vi "PH_gentec_P-Link.panel.vi"(0 "object ref":refnum<vi>, 5 "error in (no error)":errorcluster) -> (19 "error out":errorcluster)   [LabVIEW 2014, in "PH_gentec_P-Link.lvlib"]
doc: "By this VI apowermeter can be operated. \n\nThe panel is divided into the Tab Control which contains three pages and the most important elements.\nThe 1st page of the Tab Control contains the general information Range, Trigger Level, Scaling Factor (the user can set these values), Uncorrected Value and Serial Number (these are indicators). \nThe 2nd page contains everything relevant for the Statistics Mode of the powermeter. Here you can Start/Stop the statistic data collection, set the Number of Pulses, Percentage of Pulses and the Number of Samples. The Cluster 'Statistic Data' views the evaluated statistic data.\nThe 3rd page contains the rarely needed status-information of the powermeter. The string views data like Active Sensitivity, Offset, Resolution and so on.\n\nBelow the Tab Control you can see: \n - Current Value views the value that is currently being displayed on the device's screen. The correct unit is appended.\n - Powermeter views the Device State: blue means no info\n darkgreen means off\n lightgreen means operating\n yellow means error detected\n - EXIT closes the front panel (GUI), while\n - Delete Instance disconnects and removes the instance from the PCS.\n\n\nLicense Agreement for this software:\n\nCopyright (C)\nGesellschaft für Schwerionenforschung, GSI\nPlanckstr. 1\n64291 Darmstadt\nGermany\n\nContact: D.Beck@gsi.de \n\nThis program is free software; you can redistribute it and/or modify it under the terms of the GNU General Public License as published by the Free Software Foundation; either version 2 of the license, or (at your option) any later version.\n\nThis program is distributed in the hope that it will be useful, but WITHOUT ANYW ARRANTY; without even the implied warranty of MERCHANTABILITY or FITNESS FOR A PARTICULAR PURPOSE. See the GNU General License for more details (http://www.gnu.org).\n\nGesellschaft für Schwerionenforschung, GSI\nPlanckstr. 1, 64291 Darmstadt, Germany\nFor all questions and ideas contact: M.Richter@gsi.de, H.Brand@gsi.de or D.Beck@gsi.de.\nLast update: 18-DEC-2002"
uses:
  PH_gentec_P-Link.lvlib
  PH_Basics/PH_StatusHandler/PH_StatusHandler.GUI element.ctl
  PH_Basics/PH_Powermeter_BaseClass/PH_Powermeter_BaseClass.Connection.ctl
  PH_Basics/PH_Powermeter_BaseClass/PH_Powermeter_BaseClass.State.ctl
  PH_Basics/PH_Powermeter_BaseClass/PH_Powermeter_BaseClass.Head Attributes.ctl
  PH_gentec_P-Link.Head Settings.ctl
  instr.lib/Gentec-M-Link/Driver/Type Defs/gentec-M-Link.Measurement Mode.ctl
  instr.lib/Gentec-M-Link/Driver/Type Defs/gentec-M-Link.Trigger Polarity.ctl
  instr.lib/Gentec-M-Link/Driver/Type Defs/gentec-M-Link.Trigger Source.ctl
  instr.lib/Gentec-M-Link/Driver/Type Defs/gentec-M-Link.Waveform Averages.ctl
  PH_Basics/PH_Powermeter_BaseClass/PH_Powermeter_BaseClass.Energy.ctl
  PH_Basics/PH_Powermeter_BaseClass/PH_gentec_BaseClass.Head Settings.ctl
  PH_Basics/PH_Powermeter_BaseClass/PH_Powermeter_BaseClass.GUI Refs.ctl
  CS_Core/CSObj/CSObj.lvlib
  PH_Basics/PH_Common/PH_Common.lvlib
  CS_Core/CSSystem/CSSystemLib/CSSystemLib.lvlib
  PH_Basics/PH_Class/PH_Class.lvlib
  PH_Basics/PH_Powermeter_BaseClass/PH_Powermeter_BaseClass.lvlib
  instr.lib/Gentec-M-Link/gentec-M-Link - Driver.lvlib
  PH_Basics/PH_StatusHandler/PH_StatusHandler.lvlib
panel:
  in  "Tab Control":enum32{"Main", "Sets", "Information"}(tab)
  out "Power":T1={"current Value"=0.0, "unscaled"=0.0, "Scaling Factor"=1.0} {"unscaled" format="%#_6p"; "current Value" format="%#.1p"}
  out "Power evolution":dbl(graph)
  in  "Scaling Factor":dbl=1.0
  in  "Continuous":bool
  in  "get one Value":bool
  in  "Averages":T2 items=["None", "2", "4", "8", "16", "32", "64", "128"]
  in  "Range":u32(ring) items=["Scale 1", "Scale 2", "Scale 3"]
  in  "Set Auto Range":bool
  in  "Wavelength":u32 caption="nm"
  in  "Trigger Source":T3 items=["Internal", "External"]
  in  "Trigger Polarity":T4 items=["Falling Edge", "Rising Edge"]
  in  "Trigger Level":dbl caption="%"
  out "Current Settings":T5={"Trigger Level"=0.0, "Wavelength"=1, "Range"=0}
  out "Wanted Settings":T5={"Trigger Level"=0.0, "Wavelength"=1, "Range"=0}
  out "Wanted Head Settings":T6 {"Waveform Averages" items=["None", "2", "4", "8", "16", "32", "64", "128"]; "Trigger Source" items=["Internal", "External"]; "Trigger Polarity" items=["Falling Edge", "Rising Edge"]; "Measurement Mode" items=["other Mode", "Energymode"]}
  out "Current Head Settings":T6 {"Waveform Averages" items=["None", "2", "4", "8", "16", "32", "64", "128"]; "Trigger Source" items=["Internal", "External"]; "Trigger Polarity" items=["Falling Edge", "Rising Edge"]; "Measurement Mode" items=["other Mode", "Energymode"]}
  out "Connection":T8
  out "VISA resource":refnum<visa-resource-name>
  out "Head Attributes":T10={"Instrument Type"="---", "Head Version"="---", "Head Name"="---", "Serial Number"="---", "Firmware"="---", "Sensor Type"="---", "MinimumRange"=0, "Maximum Range"=0, "Min Wavelength"=-1, "Max Wavelength"=-1}
  out "PSDB Status":u32(colorbox)=6618880 caption="PSDB"
  out "Status":T11 caption="Powermeter"
  in  "Delete":bool
  in  "Exit":bool
  # "PCS"
  # "3.40"
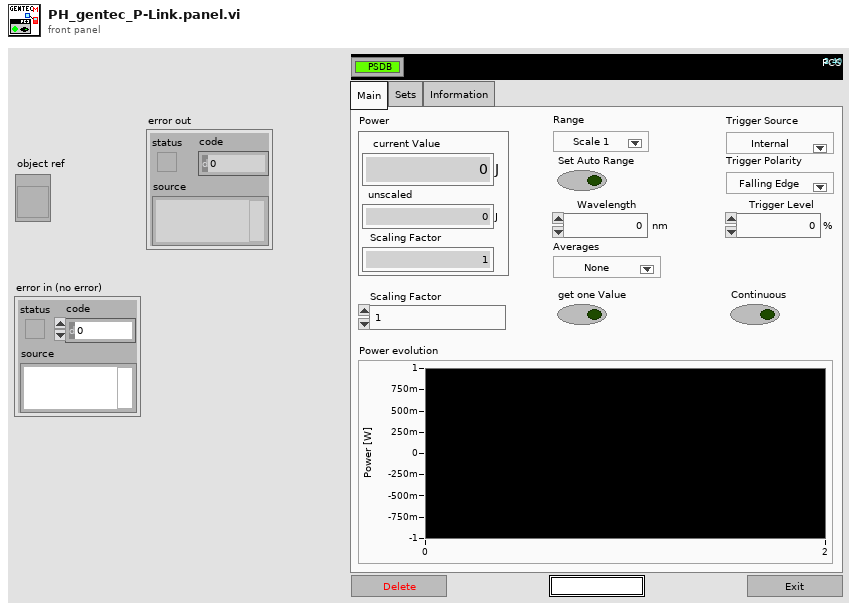
[diagram p1: front panel]
types:
  T1 = typedef "PH_Powermeter_BaseClass.lvlib/PH_Powermeter_BaseClass.Energy.ctl" = cluster{"current Value":dbl, "unscaled":dbl, "Scaling Factor":dbl}
  T2 = typedef "gentec-M-Link - Driver.lvlib/gentec-M-Link.Waveform Averages.ctl" = u16
  T3 = typedef "gentec-M-Link - Driver.lvlib/gentec-M-Link.Trigger Source.ctl" = u16
  T4 = typedef "gentec-M-Link - Driver.lvlib/gentec-M-Link.Trigger Polarity.ctl" = u16
  T5 = typedef "PH_Powermeter_BaseClass.lvlib/PH_gentec_BaseClass.Head Settings.ctl" = cluster{"Trigger Level":dbl, "Wavelength":u32, "Range":u32}
  T6 = typedef "PH_gentec_P-Link.lvlib/PH_gentec_P-Link.Head Settings.ctl" = cluster{"Measurement Mode":T7, "Enable Anticipation":bool, "Set Auto Range":bool, "Block Signal":bool, "Set Head Attenuator":bool, "Enable SSE":bool, "Trigger Polarity":T4, "Trigger Source":T3, "Waveform Averages":T2, "Set Zero":i32, "Current Measurement":i32, "Start Data Flow":bool}
  T7 = typedef "gentec-M-Link - Driver.lvlib/gentec-M-Link.Measurement Mode.ctl" = u16
  T8 = typedef "PH_Powermeter_BaseClass.lvlib/PH_Powermeter_BaseClass.Connection.ctl" = cluster{"failed checks":i8, "Timeout":bool, "Data read":string, "Failure":bool, "Error":bool, "State":T9}
  T9 = typedef "PH_Powermeter_BaseClass.lvlib/PH_Powermeter_BaseClass.State.ctl" = enum32{"off", "operating", "opened", "checked", "connected", "Sets to change", "running"}
  T10 = typedef "PH_Powermeter_BaseClass.lvlib/PH_Powermeter_BaseClass.Head Attributes.ctl" = cluster{"Instrument Type":string, "Head Version":string, "Head Name":string, "Serial Number":string, "Firmware":string, "Sensor Type":string, "MinimumRange":u32, "Maximum Range":u32, "Min Wavelength":i32, "Max Wavelength":i32}
  T11 = typedef "PH_StatusHandler.lvlib/PH_StatusHandler.GUI element.ctl" = u16
  T12 = typedef "PH_Powermeter_BaseClass.lvlib/PH_Powermeter_BaseClass.GUI Refs.ctl" = cluster{"Head Attributes":refnum<vi>, "Energy":refnum<vi>, "Connection":refnum<vi>, "VISA Resource":refnum<vi>, "Energy evolution":refnum<vi>, "Scaling Factor":refnum<vi>, "Range":refnum<vi>, "Wavelength":refnum<vi>, "Trigger Level":refnum<vi>, "Wanted Settings":refnum<vi>, "Current Settings":refnum<vi>}
  T13 = typedef "PH_gentec_P-Link.lvlib/PH_gentec_P-Link.i attribute.ctl" = cluster{"GUI References":cluster{"Wanted Head Settings":refnum<vi>, "Current Head Settings":refnum<vi>, "Set Auto Range":refnum<vi>, "Trigger Polarity":refnum<vi>, "Trigger Source":refnum<vi>, "Waveform Averages":refnum<vi>, "Continuous":refnum<vi>, "get one Value":refnum<vi>}, "Wanted Head Settings":T6, "Current Head Settings":T6}
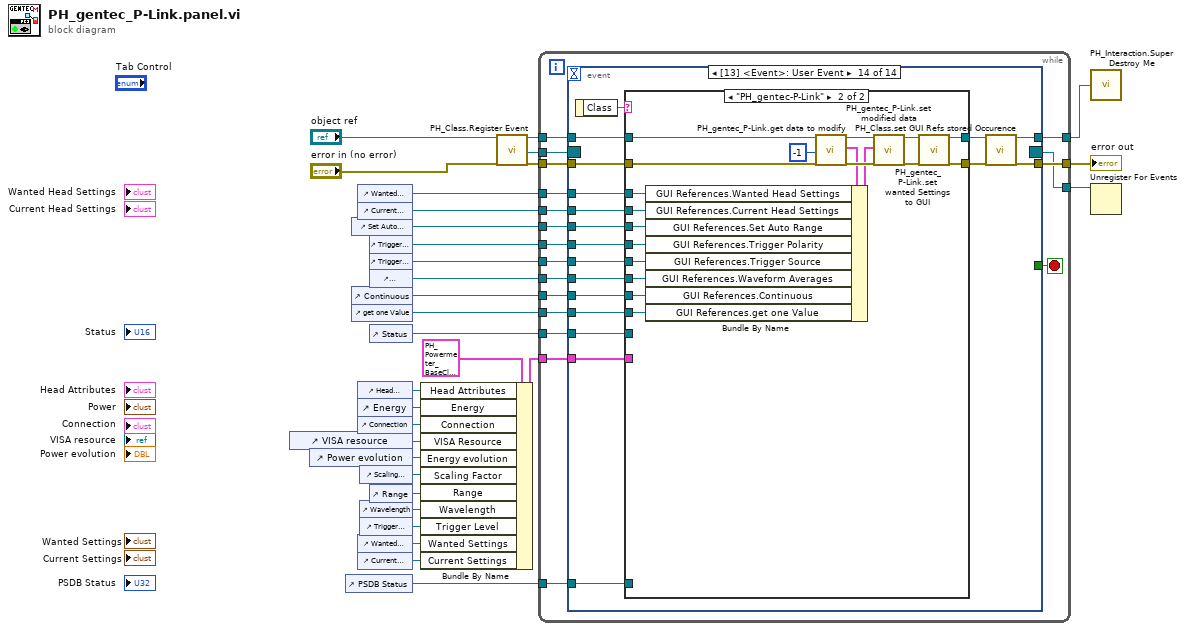
[diagram p0: block diagram]
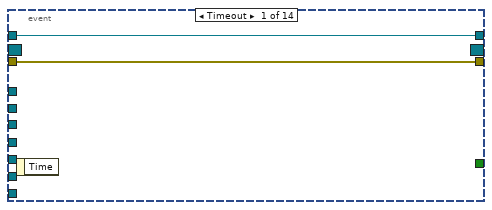
[diagram p2: hidden frame]
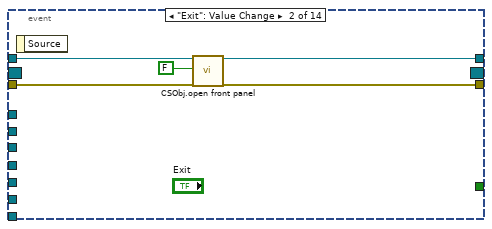
[diagram p3: hidden frame]
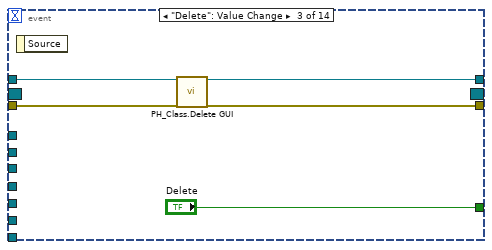
[diagram p4: hidden frame]
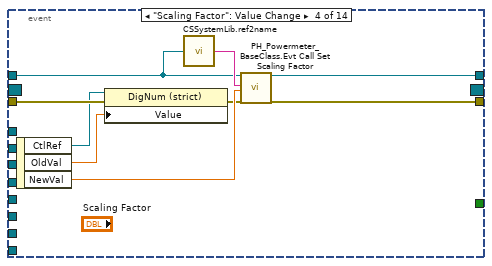
[diagram p5: hidden frame]
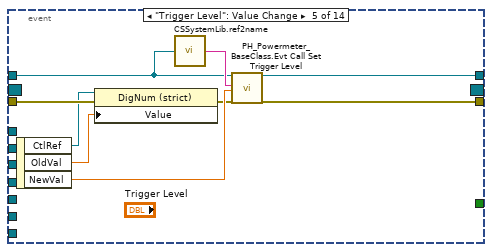
[diagram p6: hidden frame]
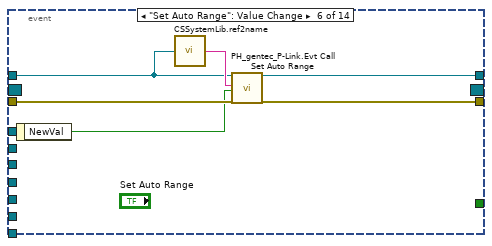
[diagram p7: hidden frame]
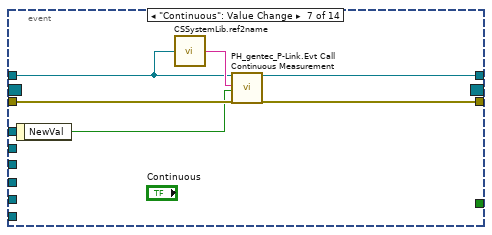
[diagram p8: hidden frame]
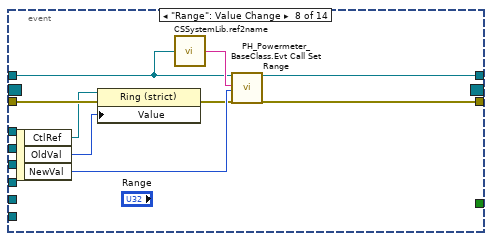
[diagram p9: hidden frame]
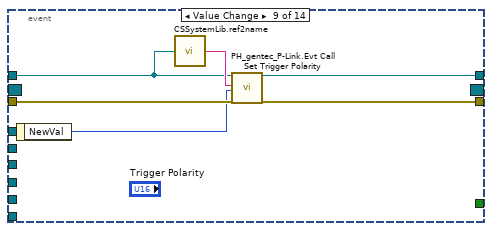
[diagram p10: hidden frame]
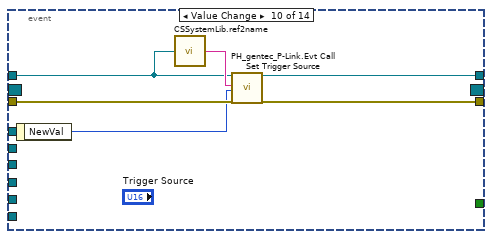
[diagram p11: hidden frame]
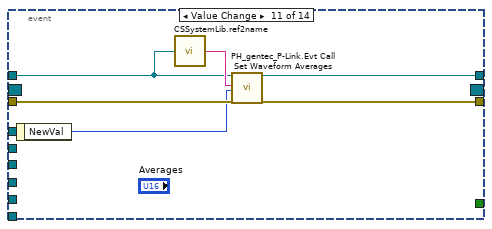
[diagram p12: hidden frame]
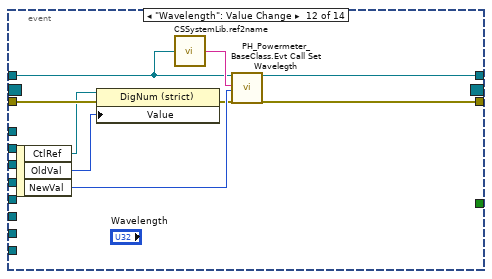
[diagram p13: hidden frame]
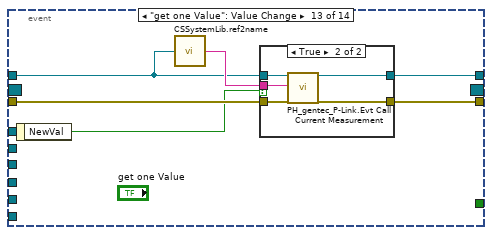
[diagram p14: hidden frame]
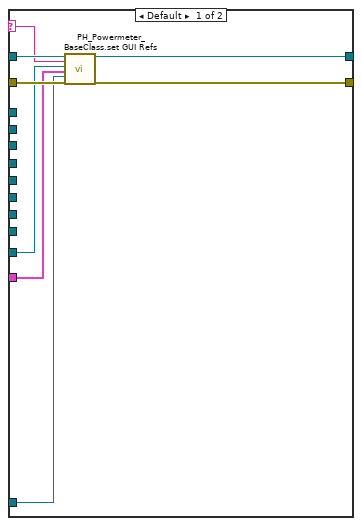
[diagram p16: hidden frame]
diagram:
  n1 = control-ref of="VISA resource"() -> (w12:refnum<vi>)
  n2 = control-ref of="Power evolution"() -> (w8:refnum<vi>)
  n3 = control-ref of="PSDB Status"() -> (w18:refnum<vi>)
  n4 = control-ref of="Set Auto Range"() -> (w24:refnum<vi>)
  n5 = control-ref of="Continuous"() -> (w20:refnum<vi>)
  n6 = control-ref of="get one Value"() -> (w19:refnum<vi>)
  n7 = control-ref of="Wanted Head Settings"() -> (w2:refnum<vi>)
  n8 = control-ref of="Current Head Settings"() -> (w1:refnum<vi>)
  n9 = control-ref of="Head Attributes"() -> (w10:refnum<vi>)
  n10 = control-ref of="Energy"() -> (w13:refnum<vi>)
  n11 = control-ref of="Connection"() -> (w11:refnum<vi>)
  n12 = control-ref of="Wanted Settings"() -> (w4:refnum<vi>)
  n13 = control-ref of="Current Settings"() -> (w3:refnum<vi>)
  n14 = control-ref of="Scaling Factor"() -> (w9:refnum<vi>)
  n15 = control-ref of="Wavelength"() -> (w6:refnum<vi>)
  n16 = control-ref of="Trigger Level"() -> (w5:refnum<vi>)
  n17 = control-ref of="Trigger Polarity"() -> (w23:refnum<vi>)
  n18 = control-ref of="Trigger Source"() -> (w22:refnum<vi>)
  n19 = control-ref of="Waveform Averages"() -> (w21:refnum<vi>)
  n20 = control-ref of="Status"() -> (w25:refnum<vi>)
  n21 = control-ref of="Range"() -> (w7:refnum<vi>)
  n22 = Bundle By Name(cluster=T12 {"Head Attributes"=refnum, "Energy"=refnum, "Connection"=refnum, "VISA Resource"=refnum, "Energy evolution"=refnum, "Scaling Factor"=refnum, "Range"=refnum, "Wavelength"=refnum, "Trigger Level"=refnum, "Wanted Settings"=refnum, "Current Settings"=refnum} ("Powermeter Base Class GUI References"), "Head Attributes"=w10, "Energy"=w13, "Connection"=w11, "VISA Resource"=w12, "Energy evolution"=w8, "Scaling Factor"=w9, "Range"=w7, "Wavelength"=w6, "Trigger Level"=w5, "Wanted Settings"=w4, "Current Settings"=w3) -> (w14:T12)
  n23 = call "PH_Class.Register Event.vi"("i ref in"="object ref", "error in (no error)"="error in (no error)") -> ("i ref out"=w29:refnum<vi>, "Event Registration Refnum"=w27:refnum<event-registration>, "error out"=w28:errorcluster)  [unwired: 15 in]
  n24 = while {
    tunnel: w29 -> [w46]
    tunnel: [w45] -> w30
    tunnel: w28 -> [w48]
    tunnel: [w47] -> w31
    tunnel: w27 -> [w44]
    tunnel: [w43] -> w26
    tunnel: w25 -> [w42]
    tunnel: w2 -> [w41]
    tunnel: w1 -> [w40]
    tunnel: w24 -> [w39]
    tunnel: w23 -> [w38]
    tunnel: w22 -> [w37]
    tunnel: w21 -> [w36]
    tunnel: w20 -> [w35]
    tunnel: w19 -> [w34]
    tunnel: w18 -> [w33]
    tunnel: w14 -> [w32]
    stop <- w49 stop-if-true
    n25 = event shown="[13] <Event>: User Event" {
      selector: w44 -> [_ _ _ _ _ _ _ _ _ _ _ _ _ _]
      dyn-events: [_ _ _ _ _ _ _ _ _ _ _ _ _ _] -> w43
      timeout: _ -> [_ _ _ _ _ _ _ _ _ _ _ _ _ _]
      tunnel: [_ _ "Delete" _ _ _ _ _ _ _ _ _ _ _] -> w49
      tunnel: w46 -> [w50 w56 w59 w65 w74 w81 w87 w96 w102 w108 w114 w123 w129 w158]
      tunnel: w48 -> [w51 w54 w60 w69 w78 w84 w90 w99 w105 w111 w117 w126 w132 w157]
      tunnel: [w51 w53 w57 w68 w77 w83 w89 w98 w104 w110 w116 w125 w131 w142] -> w47
      tunnel: [w50 w52 w58 w70 w79 w85 w91 w100 w106 w112 w118 w127 w133 w143] -> w45
      tunnel: w42 -> [_ _ _ _ _ _ _ _ _ _ _ _ _ w156]
      tunnel: w41 -> [_ _ _ _ _ _ _ _ _ _ _ _ _ w155]
      tunnel: w40 -> [_ _ _ _ _ _ _ _ _ _ _ _ _ w154]
      tunnel: w39 -> [_ _ _ _ _ _ _ _ _ _ _ _ _ w153]
      tunnel: w38 -> [_ _ _ _ _ _ _ _ _ _ _ _ _ w152]
      tunnel: w37 -> [_ _ _ _ _ _ _ _ _ _ _ _ _ w151]
      tunnel: w36 -> [_ _ _ _ _ _ _ _ _ _ _ _ _ w150]
      tunnel: w35 -> [_ _ _ _ _ _ _ _ _ _ _ _ _ w149]
      tunnel: w34 -> [_ _ _ _ _ _ _ _ _ _ _ _ _ w148]
      tunnel: w33 -> [_ _ _ _ _ _ _ _ _ _ _ _ _ w146]
      tunnel: w32 -> [_ _ _ _ _ _ _ _ _ _ _ _ _ w141]
      event Timeout {
        n26 = event-data() -> ()  [unwired: 1 in, 1 out]
      }
      event "Exit": Value Change {
        n27 = event-data() -> ()  [unwired: 1 in, 1 out]
        n28 = call "CSObj.open front panel.vi"("i ref in"=w56, "frontPanelOpen"=FALSE ("front panel open"), "error in (no error)"=w54) -> ("i ref out"=w52:refnum<vi>, "error out"=w53:errorcluster)  [unwired: 15 in]
      }
      event "Delete": Value Change {
        n29 = event-data() -> ()  [unwired: 1 in, 1 out]
        n30 = call "PH_Class.Delete GUI.vi"("VI in"=w59, "error in (no error)"=w60) -> ("VI out"=w58:refnum<vi>, "error out"=w57:errorcluster)  [unwired: 16 in]
      }
      event "Scaling Factor": Value Change {
        n31 = event-data() -> ("CtlRef"=w63:refnum<vi>, "OldVal"=w62:dbl, "NewVal"=w67:dbl)  [unwired: 1 in]
        n32 = property class="DigNum (strict)"(reference=w63, error in=w69, "Value"=w62) -> (error out=w64:errorcluster)  [unwired: 1 out]
        n33 = call "CSSystemLib.ref2name.vi"("obj refnum"=w65) -> ("name"=w66:string)
        n34 = call "PH_Powermeter_BaseClass.Evt Call Set Scaling Factor.vi"("i ref in"=w65, "Instance"=w66, "Scaling Factor"=w67, "error in (no error)"=w64) -> ("i ref out"=w70:refnum<vi>, "error out"=w68:errorcluster)  [unwired: 14 in]
      }
      event "Trigger Level": Value Change {
        n35 = event-data() -> ("CtlRef"=w72:refnum<vi>, "OldVal"=w71:dbl, "NewVal"=w76:dbl)  [unwired: 1 in]
        n36 = property class="DigNum (strict)"(reference=w72, error in=w78, "Value"=w71) -> (error out=w73:errorcluster)  [unwired: 1 out]
        n37 = call "CSSystemLib.ref2name.vi"("obj refnum"=w74) -> ("name"=w75:string)
        n38 = call "PH_Powermeter_BaseClass.Evt Call Set Trigger Level.vi"("i ref in"=w74, "Instance"=w75, "Scaling Factor"=w76, "error in (no error)"=w73) -> ("i ref out"=w79:refnum<vi>, "error out"=w77:errorcluster)  [unwired: 14 in]
      }
      event "Set Auto Range": Value Change {
        n39 = event-data() -> ("NewVal"=w80:bool)  [unwired: 1 in]
        n40 = call "CSSystemLib.ref2name.vi"("obj refnum"=w81) -> ("name"=w82:string)
        n41 = call "PH_gentec_P-Link.Evt Call Set Auto Range.vi"("i ref in"=w81, "Instance"=w82, "Set Auto Range"=w80, "error in (no error)"=w84) -> ("i ref out"=w85:refnum<vi>, "error out"=w83:errorcluster)  [unwired: 14 in]
      }
      event "Continuous": Value Change {
        n42 = event-data() -> ("NewVal"=w86:bool)  [unwired: 1 in]
        n43 = call "CSSystemLib.ref2name.vi"("obj refnum"=w87) -> ("name"=w88:string)
        n44 = call "PH_gentec_P-Link.Evt Call Continuous Measurement.vi"("i ref in"=w87, "Instance"=w88, "Continuous Measurement?"=w86, "error in (no error)"=w90) -> ("i ref out"=w91:refnum<vi>, "error out"=w89:errorcluster)  [unwired: 14 in]
      }
      event "Range": Value Change {
        n45 = event-data() -> ("CtlRef"=w93:refnum<vi>, "OldVal"=w92:u32, "NewVal"=w95:u32)  [unwired: 1 in]
        n46 = property class="Ring (strict)"(reference=w93, error in=w99, "Value"=w92) -> (error out=w94:errorcluster)  [unwired: 1 out]
        n47 = call "CSSystemLib.ref2name.vi"("obj refnum"=w96) -> ("name"=w97:string)
        n48 = call "PH_Powermeter_BaseClass.Evt Call Set Range.vi"("i ref in"=w96, "Instance"=w97, "Range"=w95, "error in (no error)"=w94) -> ("i ref out"=w100:refnum<vi>, "error out"=w98:errorcluster)  [unwired: 14 in]
      }
      event Value Change {
        n49 = event-data() -> ("NewVal"=w101:T4)  [unwired: 1 in]
        n50 = call "CSSystemLib.ref2name.vi"("obj refnum"=w102) -> ("name"=w103:string)
        n51 = call "PH_gentec_P-Link.Evt Call Set Trigger Polarity.vi"("i ref in"=w102, "Instance"=w103, "Trigger Polarity"=w101, "error in (no error)"=w105) -> ("i ref out"=w106:refnum<vi>, "error out"=w104:errorcluster)  [unwired: 14 in]
      }
      event Value Change {
        n52 = event-data() -> ("NewVal"=w107:T3)  [unwired: 1 in]
        n53 = call "CSSystemLib.ref2name.vi"("obj refnum"=w108) -> ("name"=w109:string)
        n54 = call "PH_gentec_P-Link.Evt Call Set Trigger Source.vi"("i ref in"=w108, "Instance"=w109, "Trigger Source Source"=w107, "error in (no error)"=w111) -> ("i ref out"=w112:refnum<vi>, "error out"=w110:errorcluster)  [unwired: 14 in]
      }
      event Value Change {
        n55 = event-data() -> ("NewVal"=w113:T2)  [unwired: 1 in]
        n56 = call "CSSystemLib.ref2name.vi"("obj refnum"=w114) -> ("name"=w115:string)
        n57 = call "PH_gentec_P-Link.Evt Call Set Waveform Averages.vi"("i ref in"=w114, "Instance"=w115, "Waveform Averages"=w113, "error in (no error)"=w117) -> ("i ref out"=w118:refnum<vi>, "error out"=w116:errorcluster)  [unwired: 14 in]
      }
      event "Wavelength": Value Change {
        n58 = event-data() -> ("CtlRef"=w120:refnum<vi>, "OldVal"=w119:u32, "NewVal"=w122:u32)  [unwired: 1 in]
        n59 = property class="DigNum (strict)"(reference=w120, error in=w126, "Value"=w119) -> (error out=w121:errorcluster)  [unwired: 1 out]
        n60 = call "CSSystemLib.ref2name.vi"("obj refnum"=w123) -> ("name"=w124:string)
        n61 = call "PH_Powermeter_BaseClass.Evt Call Set Wavelegth.vi"("i ref in"=w123, "Instance"=w124, "Scaling Factor"=w122, "error in (no error)"=w121) -> ("i ref out"=w127:refnum<vi>, "error out"=w125:errorcluster)  [unwired: 14 in]
      }
      event "get one Value": Value Change {
        n62 = event-data() -> ("NewVal"=w128:bool)  [unwired: 1 in]
        n63 = call "CSSystemLib.ref2name.vi"("obj refnum"=w129) -> ("name"=w130:string)
        n64 = case shown="True" w128 {
          tunnel: [w135 w140] -> w133
          tunnel: w132 -> [w134 w139]
          tunnel: [w134 w138] -> w131
          tunnel: w130 -> [_ w137]
          tunnel: w129 -> [w135 w136]
          frame False {
          }
          frame True {
            n65 = call "PH_gentec_P-Link.Evt Call Current Measurement.vi"("i ref in"=w136, "Instance"=w137, "error in (no error)"=w139) -> ("i ref out"=w140:refnum<vi>, "error out"=w138:errorcluster)  [unwired: 15 in]
          }
        }
      }
      event User Event {
        n66 = event-data() -> ("Class"=w147:string)  [unwired: 1 in]
        n67 = case shown="\"PH_gentec-P-Link\"" w147 {
          selector: w147 -> [w164 _]
          tunnel: w158 -> [w165 w181]
          tunnel: w157 -> [w166 w180]
          tunnel: [w162 w169] -> w145
          tunnel: [w161 w168] -> w144
          tunnel: w156 -> [w163 _]
          tunnel: w155 -> [_ w179]
          tunnel: w154 -> [_ w178]
          tunnel: w153 -> [_ w177]
          tunnel: w152 -> [_ w176]
          tunnel: w151 -> [_ w175]
          tunnel: w150 -> [_ w174]
          tunnel: w149 -> [_ w173]
          tunnel: w148 -> [_ w172]
          tunnel: w146 -> [w160 _]
          tunnel: w141 -> [w159 _]
          frame Default {
            n68 = call "PH_Powermeter_BaseClass.set GUI Refs.vi"("VI in"=w165, "Class"=w164, "Status GUI Reference"=w163, "Powermeter Base Class GUI References"=w159, "PSDB Status GUI Reference"=w160, "error in (no error)"=w166) -> ("VI out"=w162:refnum<vi>, "error out"=w161:errorcluster)  [unwired: 12 in]
          }
          frame "PH_gentec-P-Link" {
            n69 = call "PH_gentec_P-Link.get data to modify.vi"("i ref in"=w181, "ms timeout (10000)"=-1, "error in (no error)"=w180) -> ("i ref out"=w185:refnum<vi>, "i attribute"=w182:T13, "error out"=w184:errorcluster)  [unwired: 13 in, 1 out]
            n70 = Bundle By Name(cluster=w182, "GUI References.Wanted Head Settings"=w179, "GUI References.Current Head Settings"=w178, "GUI References.Set Auto Range"=w177, "GUI References.Trigger Polarity"=w176, "GUI References.Trigger Source"=w175, "GUI References.Waveform Averages"=w174, "GUI References.Continuous"=w173, "GUI References.get one Value"=w172) -> (w167:T13)
            n71 = call "PH_gentec_P-Link.set modified data.vi"("i ref in"=w185, "i attribute"=w167, "error in (no error)"=w184) -> ("i ref out"=w170:refnum<vi>, "error out"=w171:errorcluster)  [unwired: 15 in]
            n72 = call "PH_gentec_P-Link.set wanted Settings to GUI.vi"("i ref in"=w170, "error in"=w171) -> ("i ref out"=w169:refnum<vi>, "error out"=w168:errorcluster)  [unwired: 16 in]
          }
        }
        n73 = call "PH_Class.set GUI Refs stored Occurence.vi"("i ref in"=w145, "error in (no error)"=w144) -> ("i ref out"=w143:refnum<vi>, "error out"=w142:errorcluster)  [unwired: 16 in]
      }
    }
  }
  "error out" <- w31
  n74 = call "PH_Interaction.Super Destroy Me.vi"("i ref out"=w30) -> ()
  n75 = Unregister For Events(event registration refnum=w26) -> ()  [unwired: 1 in, 1 out]
